vi "Read Lines from File - With Error in and Error Out - JKI.vi"(0 "file path (dialog if empty)":path, 1 "prompt":string="Choose file to read.", 5 "number of lines (all:-1)":i32=-1, 7 "start of read offset (chars.:0)":i32, 9 "[max characters per line]  (no limit:0)":i32, 11 "error in (no error)":errorcluster, 12 "convert eol? (no:F)":bool) -> (4 "new file path (Not A Path if cancelled)":path, 6 "line string":string, 8 "mark after read (chars.)":i32, 10 "EOF?":bool, 15 "error out":errorcluster)   [LabVIEW 2011]
panel:
  # "Copyright © 2006 James Kring, Inc. All rights reserved.\n\nAuthor: Philippe Guerit [philippe.guerit@jameskring.com]\n             [alternate email: PJM_LabVIEW@yahoo.com]\n\nThis library is provided \"AS IS\" ,WITHOUT WARRANTIES OR \nCONDITIONS OF ANY KIND, either express or implied.\n\nJames Kring, Inc. -- http://www.jameskring.com"
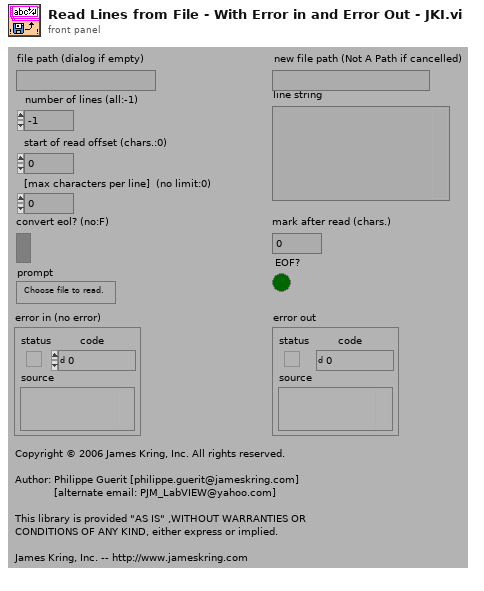
[diagram p1: front panel]
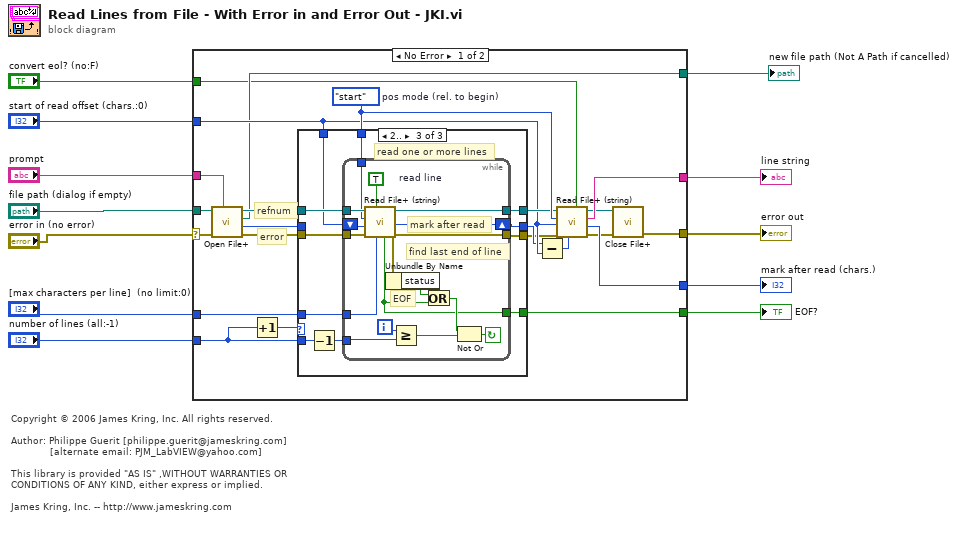
[diagram p0: block diagram]
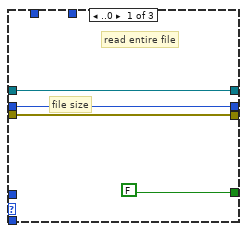
[diagram p2: hidden frame]
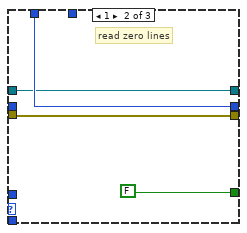
[diagram p3: hidden frame]
diagram:
  # "Copyright © 2006 James Kring, Inc. All rights reserved.\n\nAuthor: Philippe Guerit [philippe.guerit@jameskring.com]\n             [alternate email: PJM_LabVIEW@yahoo.com]\n\nThis library is provided \"AS IS\" ,WITHOUT WARRANTIES OR \nCONDITIONS OF ANY KIND, either express or implied.\n\nJames Kring, Inc. -- http://www.jameskring.com"
  n1 = case shown="No Error" "error in (no error)" {
    selector: "error in (no error)" -> [w13 w71]
    tunnel: "prompt" -> [w35 _]
    tunnel: "number of lines (all:-1)" -> [w33 _]
    tunnel: [w32 _] -> w10
    tunnel: "start of read offset (chars.:0)" -> [w29 _]
    tunnel: "[max characters per line]  (no limit:0)" -> [w26 _]
    tunnel: [w22 _] -> w7
    tunnel: "convert eol? (no:F)" -> [w21 _]
    tunnel: [w20 _] -> w5
    tunnel: [w19 _] -> w4
    tunnel: "file path (dialog if empty)" -> [w15 _]
    tunnel: [w14 w71] -> w2
    frame No Error {
      w34 = enum16{"start", "end", "current"}."start"  # pos mode (rel. to begin)
      # "error"
      # "refnum"
      n2 = call <vilib>:"Open File+.vi"("prompt"=w35, "error in (not an error)"=w13, "file path (\" \")"=w15) -> ("error out"=w27:errorcluster, "file size (bytes)"=w30:i32, "file path"=w22:path, "refnum"=w28:refnum<file>)  [unwired: 5 in]
      n3 = Increment(x=w33) -> (x+1=w25:i32)
      n4 = case shown="2.." w25 {
        tunnel: [w39 w42 w54] -> w23
        tunnel: [w38 w43 w53] -> w24
        tunnel: w33 -> [_ _ w52]
        tunnel: w26 -> [_ _ w51]
        tunnel: w27 -> [w39 w42 w50]
        tunnel: w28 -> [w37 w41 w49]
        tunnel: w29 -> [_ w43 w48]
        tunnel: w34 -> [_ _ w47]
        tunnel: w30 -> [w38 _ _]
        tunnel: [w37 w41 w46] -> w31
        tunnel: [FALSE FALSE w45] -> w32
        frame ..0 {
          # "file size"
          # "read entire file"
        }
        frame 1 {
          # "read zero lines"
        }
        frame 2.. {
          # "read one or more lines"
          n5 = Decrement(x=w52) -> (x-1=w44:i32)
          n6 = while {
            tunnel: [w56] -> w45
            tunnel: w47 -> [w61]
            tunnel: w50 -> [w63]
            tunnel: w51 -> [w64]
            tunnel: [w59] -> w54
            tunnel: w49 -> [w66]
            tunnel: [w67] -> w46
            tunnel: w44 -> [w55]
            shift-left: w48 -> [w68]
            shift-right: [w70] -> w53
            i -> [w69]
            stop <- w62 continue-if-true
            w58 = TRUE  # read line
            # "mark after read"
            # "find last end of line"
            # "EOF"
            n7 = call <vilib>:"Read File+ (string).vi"("count"=w64, "line mode (characters:F)"=w58, "error in (no error)"=w63, "pos offset (bytes:0)"=w68, "pos mode (rel. to current:2)"=w61, "refnum"=w66) -> ("error out"=w59:errorcluster, "mark after read (bytes)"=w70:i32, "dup refnum"=w67:refnum<file>, "EOF?"=w56:bool)  [unwired: 1 in, 1 out]
            n8 = Unbundle By Name(w59) -> ("status"=w57:bool)
            n9 = Greater Or Equal?(x=w69, y=w55) -> (x >= y?=w65:bool)
            n10 = Or(x=w57, y=w56) -> (x .or. y?=w60:bool)
            n11 = Not Or(1:w65, 2:w60) -> (0:w62:bool)
          }
        }
      }
      n12 = Subtract(x=w24, y=w29) -> (x-y=w18:i32)
      n13 = call <vilib>:"Read File+ (string).vi"("convert eol? (no:F)"=w21, "count"=w18, "error in (no error)"=w23, "pos offset (bytes:0)"=w29, "pos mode (rel. to current:2)"=w34, "refnum"=w31) -> ("error out"=w17:errorcluster, "mark after read (bytes)"=w20:i32, "string"=w19:string, "dup refnum"=w16:refnum<file>)  [unwired: 1 in, 1 out]
      n14 = call <vilib>:"Close File+.vi"("error in (no error)"=w17, "refnum"=w16) -> ("error out"=w14:errorcluster)  [unwired: 3 in, 2 out]
    }
    frame Error {
    }
  }
  "error out" <- w2
  "new file path (Not A Path if cancelled)" <- w7
  "line string" <- w4
  "mark after read (chars.)" <- w5
  "EOF?" <- w10
